vi "Measure.vi"(8 "error in (no error)":errorcluster, 10 "unit":T1, 11 "TemperatureSensor in":refnum<class "TemperatureSensor.lvclass">) -> (0 "error out":errorcluster, 2 "measurement":dbl, 3 "TemperatureSensor out":refnum<class "TemperatureSensor.lvclass">)   [LabVIEW 2019, in "TemperatureSensor.lvclass"]
uses:
  TemperatureSensor.lvclass
  Units.ctl
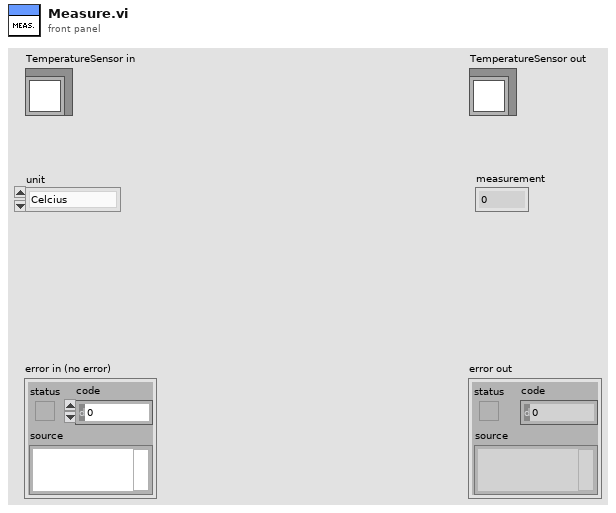
[diagram p1: front panel]
types:
  T1 = typedef "TemperatureSensor.lvclass/Units.ctl" = enum16{"Celcius", "Fahrenheit"}
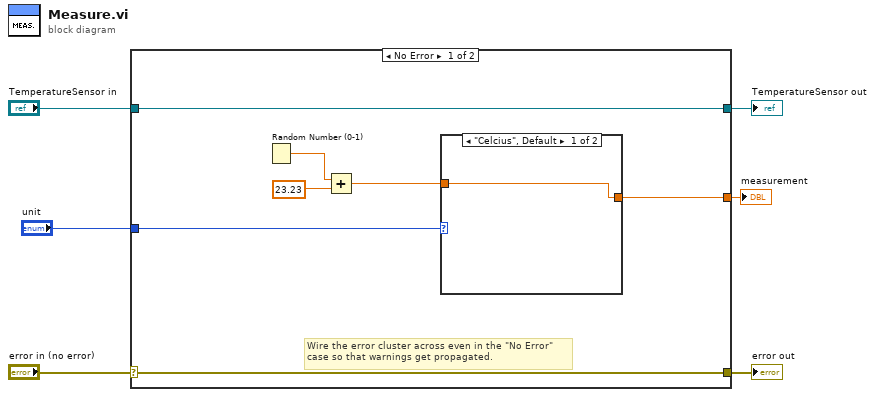
[diagram p0: block diagram]
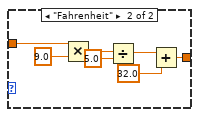
[diagram p2: hidden frame]
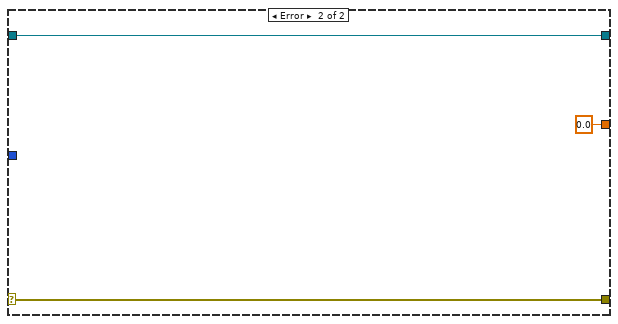
[diagram p3: hidden frame]
diagram:
  n1 = case shown="No Error" "error in (no error)" {
    selector: "error in (no error)" -> [w12 w24]
    tunnel: [w12 w24] -> w5
    tunnel: [w13 w23] -> w3
    tunnel: "TemperatureSensor in" -> [w13 w23]
    tunnel: "unit" -> [w9 _]
    tunnel: [w7 0.0] -> w1
    frame No Error {
      # "Wire the error cluster across even in the \"No Error\"\ncase so that warnings get propagated."
      n2 = Random Number (0-1)() -> (number: 0 to 1=w10:dbl)
      n3 = Add(x=w10, y=23.23) -> (x+y=w8:dbl)
      n4 = case shown="\"Celcius\", Default" w9 {
        tunnel: w8 -> [w14 w21]
        tunnel: [w14 w15] -> w7
        frame "Celcius", Default {
        }
        frame "Fahrenheit" {
          n5 = Multiply(x=w21, y=9.0) -> (x*y=w19:dbl)
          n6 = Divide(x=w19, y=5.0) -> (x/y=w17:dbl)
          n7 = Add(x=w17, y=32.0) -> (x+y=w15:dbl)
        }
      }
    }
    frame Error {
    }
  }
  "error out" <- w5
  "TemperatureSensor out" <- w3
  "measurement" <- w1
